vi "CalDataSave.vi"(2 "Data Array":cluster{"Radians":dbl[], "Sensor":dbl[]}[](array[cluster]), 3 "Save Path":path) -> (1 "File Path Out":path)   [LabVIEW 2012]
doc: "Processes the Data Array created by CgCalibrate and formats the data from the cluster of arrays into an appropriate spreadsheet. Writes to the indicated file."
uses:
  <vilib>/Utility/file.llb/Write To Spreadsheet File (DBL).vi
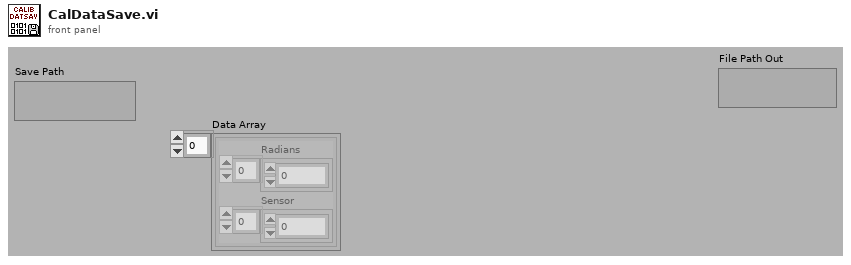
[diagram p1: front panel]
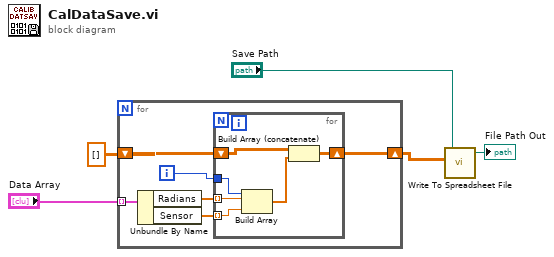
[diagram p0: block diagram]
diagram:
  n1 = for {
    tunnel: "Data Array" -> [w11] mode=indexing
    shift-right: [w6] -> w5
    shift-left: dbl[][] [] -> [w7]
    i -> [w10]
    n2 = Unbundle By Name(w11) -> ("Radians"=w9:dbl[], "Sensor"=w8:dbl[])
    n3 = for {
      tunnel: w10 -> [w17]
      tunnel: w9 -> [w16] mode=indexing
      tunnel: w8 -> [w15] mode=indexing
      shift-right: [w13] -> w6
      shift-left: w7 -> [w12]
      n4 = Build Array(w17, w16, w15) -> (w14:dbl[])
      n5 = Build Array (concatenate)(w12, w14) -> (w13:dbl[][])
    }
  }
  n6 = call-poly <vilib>:"Write To Spreadsheet File.vi"("2D data"=w5, "file path (dialog if empty)"="Save Path") -> ("new file path (Not A Path if cancelled)"=→"File Path Out":path)  [unwired: 6 in]
